vi "FTW-ZMQ-Context-Construct.vi"(11 "error in":errorcluster) -> (4 "ZeroMQ Context":refnum<class "FTW-ZMQ-Context.lvclass">, 15 "error out":errorcluster)   [LabVIEW 2014, in "FTW-ZMQ-Context.lvclass"]
uses:
  FTW-ZMQ-Context.lvclass
  FTW-ZMQ-Context.lvclass/FTW-ZMQ-Context.ctl
panel:
  # "Inputs"
  # "Outputs"
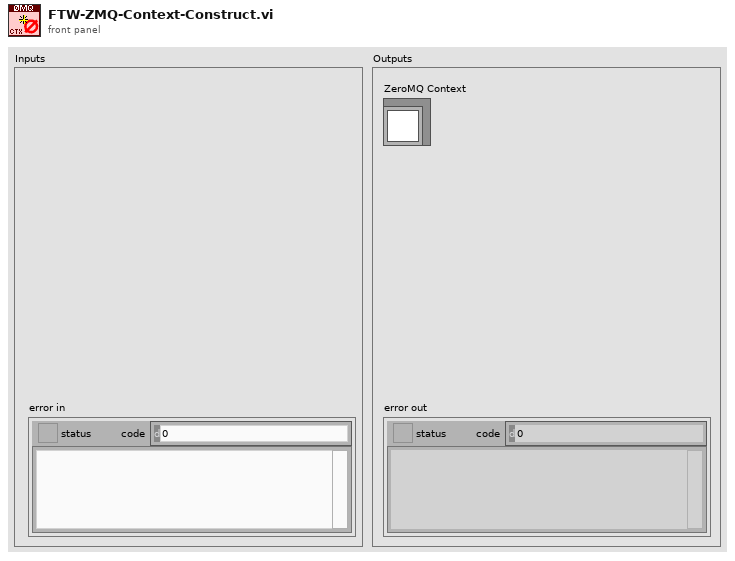
[diagram p1: front panel]
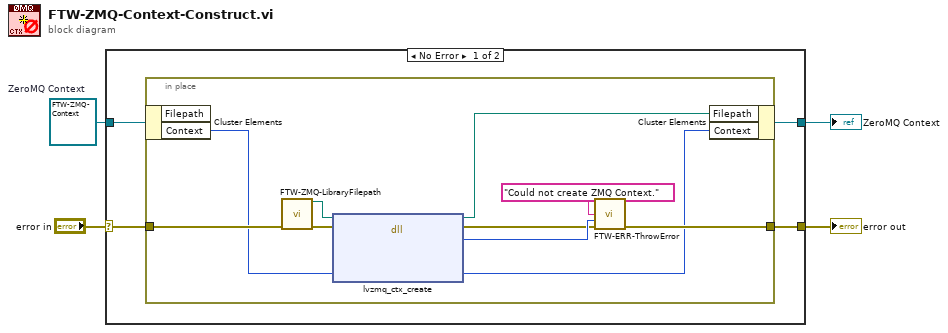
[diagram p0: block diagram]
diagram:
  w1 = refnum<class "FTW-ZMQ-Context.lvclass"> refnum  # ZeroMQ Context
  n1 = case shown="No Error" "error in" {
    selector: "error in" -> [w8 w20]
    tunnel: [w7 w20] -> w4
    tunnel: [w5 w19] -> w3
    tunnel: w1 -> [w6 w19]
    frame No Error {
      n2 = in-place {
        in-place-border: w8 -> [w18]
        in-place-border: [w13] -> w7
        n3 = in-place-cluster #1(w6) -> ("Context"=w9:u64)  [unwired: 1 out]
        n4 = call "FTW-ZMQ-LibraryFilepath.vi"("error in"=w18) -> ("FTW-ZMQ Library Filepath"=w17:path, "error out"=w16:errorcluster)  [unwired: 12 in, 1 out]
        n5 = dll-call lib="?" fn="lvzmq_ctx_create" ("zmq_labview.dll:lvzmq_init")(path in=w17, error in=w16, "Context Pointer"=w9) -> (path out=w11:path, error out=w14:errorcluster, "Return Value"=w15:i32, "Context Pointer"=w10:u64)  [unwired: 3 in]
        n6 = call "FTW-ERR-ThrowError.vi"("Error Message"="Could not create ZMQ Context.", "Error Code"=w15, "error in"=w14) -> ("error out"=w13:errorcluster)  [unwired: 12 in]
        n7 = in-place-cluster #1("Filepath"=w11, "Context"=w10) -> (w5:refnum<class "FTW-ZMQ-Context.lvclass">)
      }
    }
    frame Error {
    }
  }
  "error out" <- w4
  "ZeroMQ Context" <- w3
